vi "Command.vi"(8 "error in (no error)":errorcluster, 9 "data in":u8[](array[numeric]) format="%x", 10 "function code":u8=1 format="%x", 11 "MODBUS in":refnum<class "PL Modbus Client.lvclass">) -> (0 "error out":errorcluster, 2 "data out":u8[](array[numeric]) format="%x", 3 "MODBUS out":refnum<class "PL Modbus Client.lvclass">)   [LabVIEW 2015, in "PL Modbus Client.lvclass"]
doc: "Sends Modbus request with specified <B>function code</B> and <B>data in</B> and returns response data as <B>data out</B>. For not implemented function codes used via Modbus RTU <B>read RTU data callback</B> should be provided (default Read RTU Data.vi can be used as a template)."
uses:
  PL Modbus Client.lvclass
  PL Modbus Client.lvclass/PL Modbus Client.ctl
panel:
  out "exception":bool
  out "read buffer":string
  out "VISA locked":bool
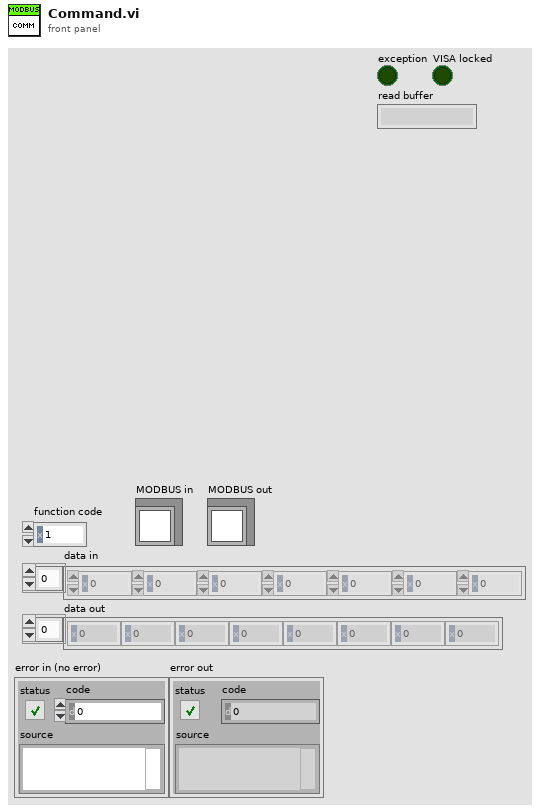
[diagram p1: front panel]
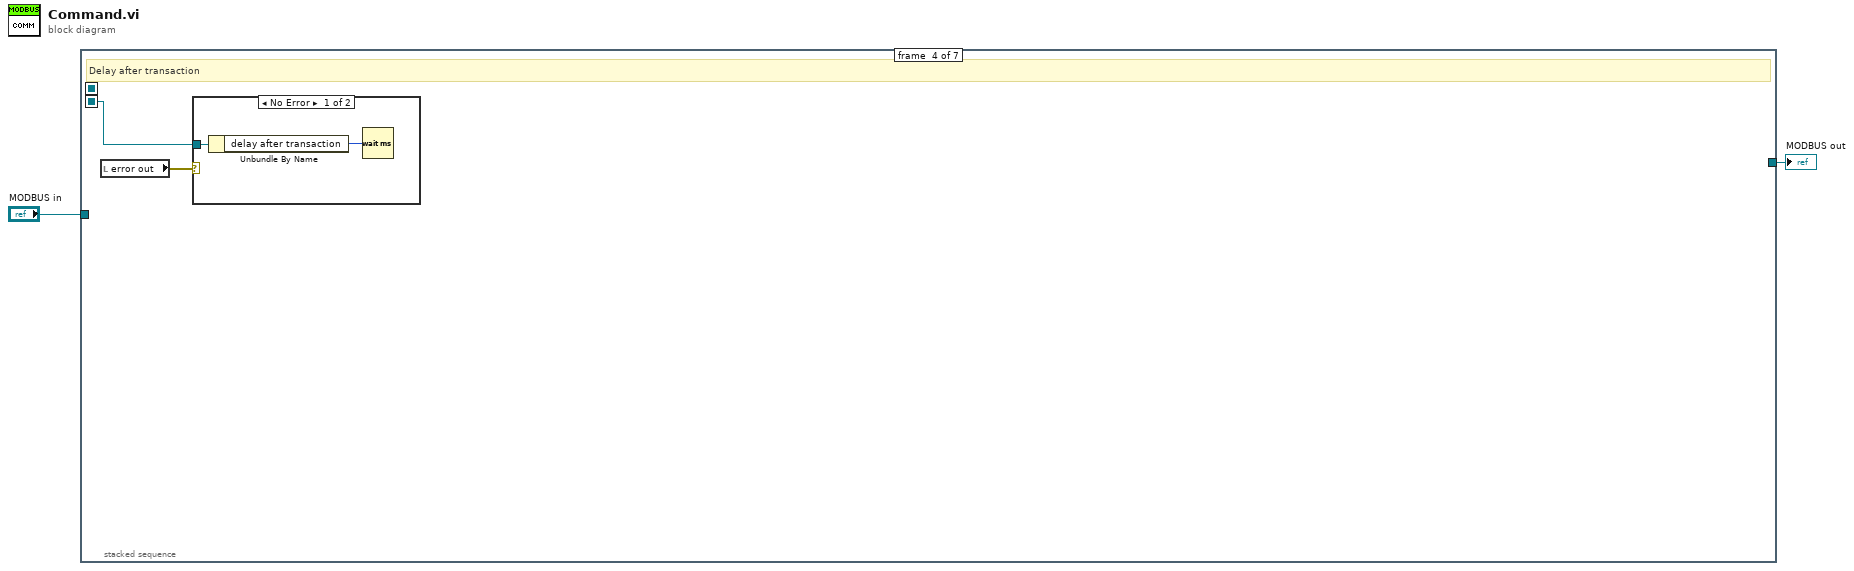
[diagram p0: block diagram]
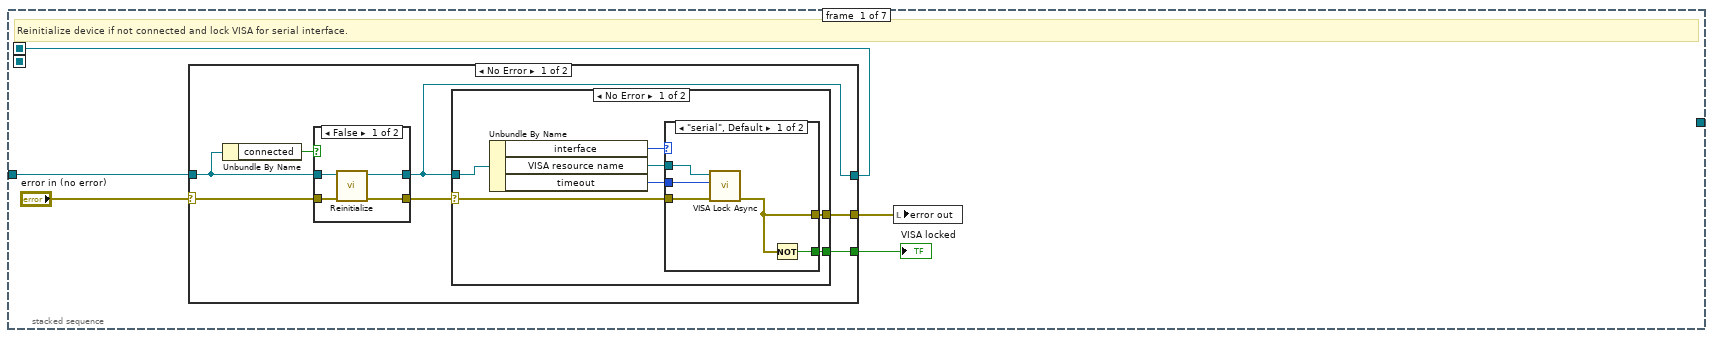
[diagram p2: hidden frame]
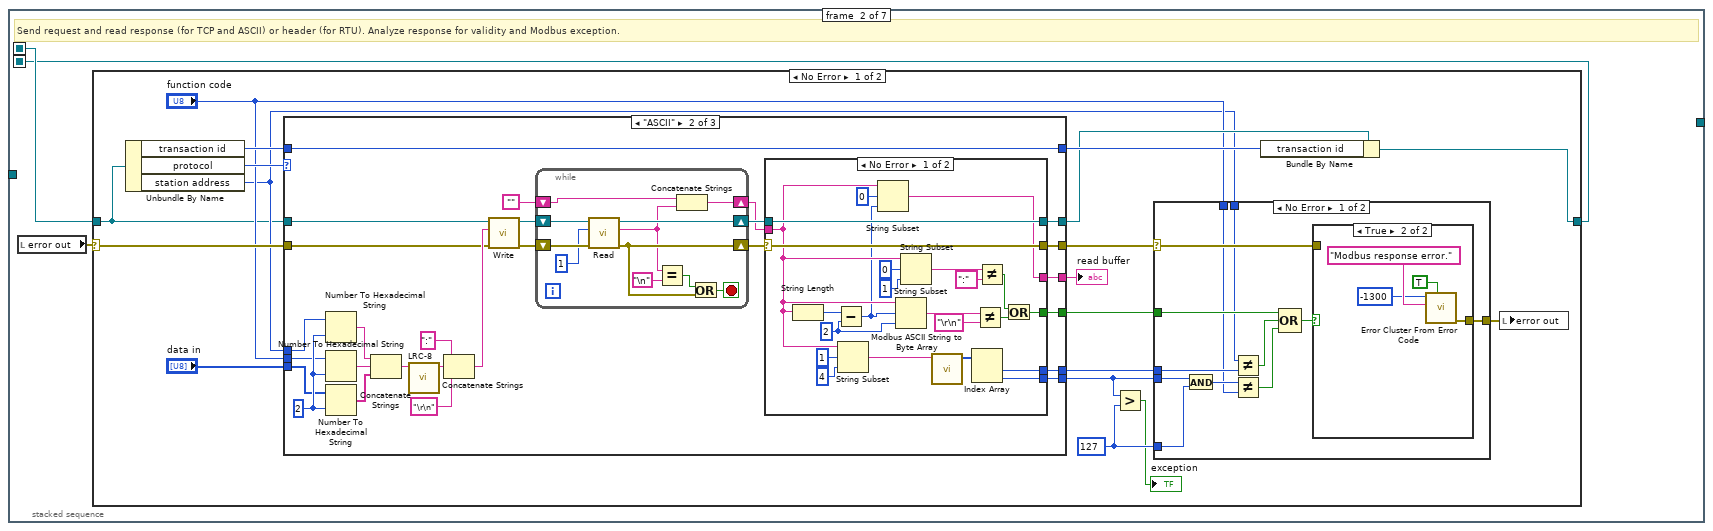
[diagram p7: hidden frame]
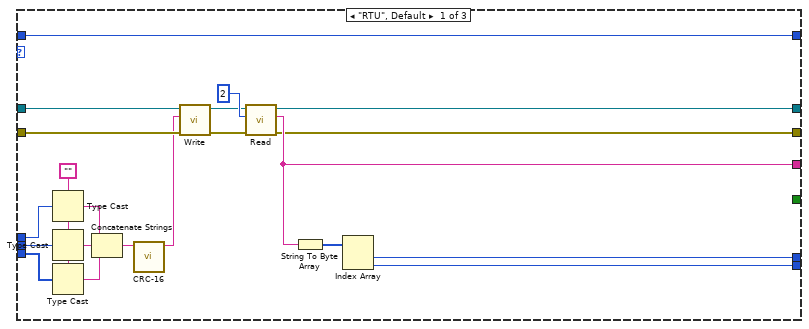
[diagram p10: hidden frame]
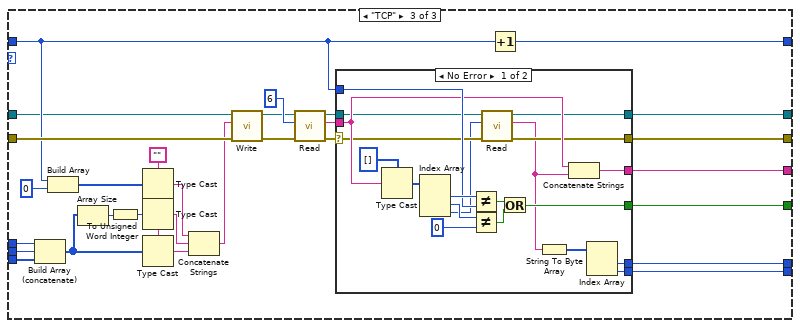
[diagram p12: hidden frame]
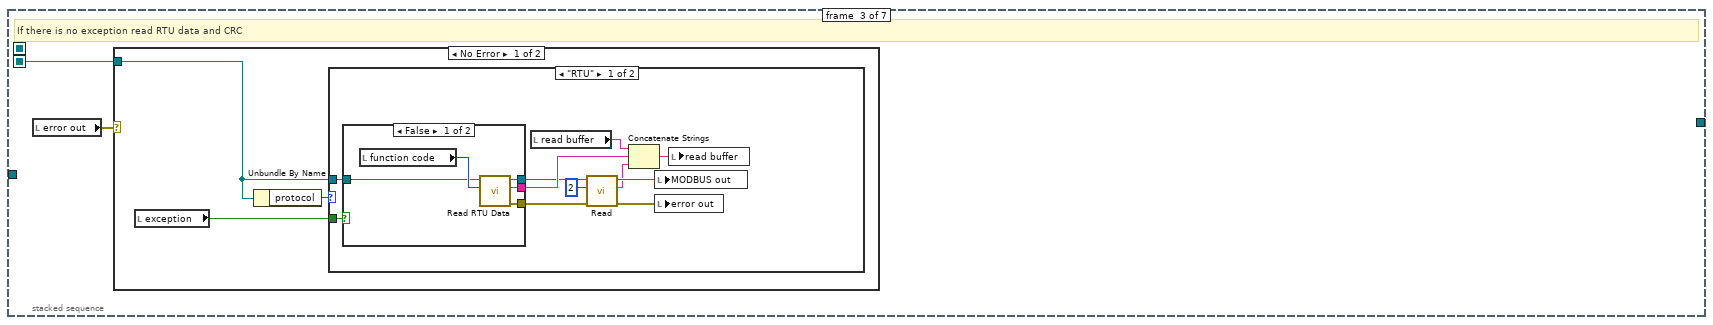
[diagram p15: hidden frame]
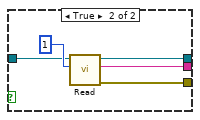
[diagram p16: hidden frame]
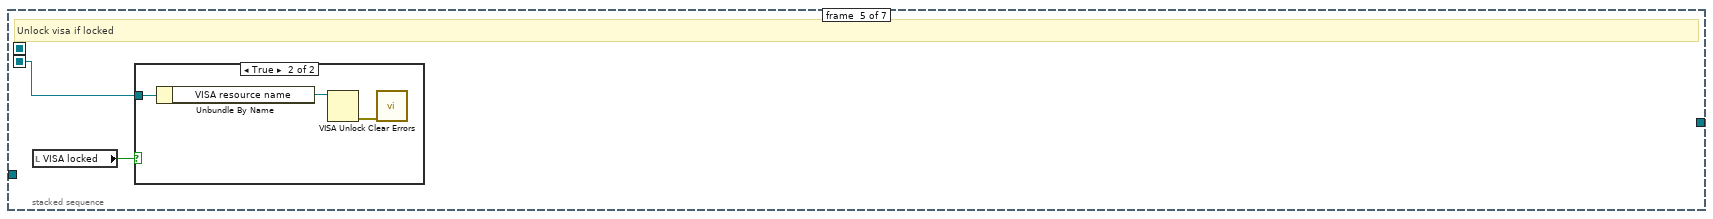
[diagram p20: hidden frame]
diagram:
  n1 = stacked-sequence {
    seq-local: [w4 _ _ _ _ _ _] -> [_ w38 _ _ _ _ _]
    seq-local: [_ w37 _ _ _ _ _] -> [_ _ w212 w239 w242 w247 w264]
    tunnel: [_ _ _ _ _ _ w263] -> w2
    tunnel: "MODBUS in" -> [w3 _ _ _ _ _ _]
    frame #0 {
      # "Reinitialize device if not connected and lock VISA for serial interface."
      n2 = case shown="No Error" "error in (no error)" {
        selector: "error in (no error)" -> [w9 w35]
        tunnel: [w14 _] -> w7
        tunnel: [w13 w35] -> w6
        tunnel: w3 -> [w11 w36]
        tunnel: [w8 w36] -> w4
        frame No Error {
          n3 = Unbundle By Name(w11) -> ("connected"=w12:bool)
          n4 = case shown="False" w12 {
            tunnel: w11 -> [w18 w20]
            tunnel: [w17 w20] -> w8
            tunnel: w9 -> [w15 w19]
            tunnel: [w16 w19] -> w10
            frame False {
              n5 = call "Reinitialize.vi"("error in (no error)"=w15, "MODBUS in"=w18) -> ("error out"=w16:errorcluster, "MODBUS out"=w17:refnum<class "PL Modbus Client.lvclass">)  [unwired: 8 in]
            }
            frame True {
            }
          }
          n6 = case shown="No Error" w10 {
            selector: w10 -> [w21 w34]
            tunnel: w8 -> [w26 _]
            tunnel: [w23 _] -> w14
            tunnel: [w22 w34] -> w13
            frame No Error {
              n7 = Unbundle By Name(w26) -> ("interface"=w27:enum16{"serial", "network"}, "VISA resource name"=w25:refnum<visa-resource-name>, "timeout"=w24:u32)
              n8 = case shown="\"serial\", Default" w27 {
                tunnel: w25 -> [w32 _]
                tunnel: w24 -> [w31 _]
                tunnel: [w30 _] -> w23
                tunnel: [w29 w33] -> w22
                tunnel: w21 -> [w28 w33]
                frame "serial", Default {
                  n9 = call <vilib>:"VISA Lock Async.vi"("error in (no error)"=w28, "timeout (0)"=w31, "VISA resource name"=w32) -> ("error out"=w29:errorcluster)  [unwired: 6 in, 2 out]
                  n10 = Not(x=w29) -> (.not. x?=w30:bool)
                }
                frame "network" {
                }
              }
            }
            frame Error {
            }
          }
        }
        frame Error {
        }
      }
      "VISA locked" <- w7
      n11 = local write "error out"(w6) -> ()
    }
    frame #1 {
      # "Send request and read response (for TCP and ASCII) or header (for RTU). Analyze response for validity and Modbus exception."
      n12 = local read "error out"() -> (w39:errorcluster)
      n13 = case shown="No Error" w39 {
        selector: w39 -> [w47 _]
        tunnel: w38 -> [w41 w211]
        tunnel: [w40 w211] -> w37
        frame No Error {
          w51 = u8 127
          n14 = Unbundle By Name(w41) -> ("transaction id"=w56:u16, "protocol"=w46:enum16{"RTU", "ASCII", "TCP"}, "station address"=w42:u8)
          n15 = case shown="\"ASCII\"" w46 {
            tunnel: w47 -> [w80 w98 w166]
            tunnel: [w77 w122 w187] -> w55
            tunnel: [w92 w113 w186] -> w45
            tunnel: [w96 w123 w188] -> w57
            tunnel: w56 -> [w96 w123 w161]
            tunnel: [w95 w119 w185] -> w53
            tunnel: [w94 w118 w184] -> w52
            tunnel: [_ w121 w183] -> w54
            tunnel: [w91 w120 w182] -> w48
            tunnel: w41 -> [w78 w97 w160]
            tunnel: "data in" -> [w82 w100 w168]
            tunnel: "function code" -> [w84 w102 w165]
            tunnel: w42 -> [w83 w101 w164]
            frame "RTU", Default {
              w85 = ""
              n16 = Type Cast(type=w85, x=w83) -> (*(type *) &x=w86:string)
              n17 = Type Cast(type=w85, x=w84) -> (*(type *) &x=w87:string)
              n18 = Type Cast(type=w85, x=w82) -> (*(type *) &x=w88:string)
              n19 = Concatenate Strings(w86, w87, w88) -> (w89:string)
              n20 = call "CRC-16.vi"("string"=w89) -> ("string with CRC-16"=w79:string)  [unwired: 9 in, 1 out]
              n21 = call "Write.vi"("error in (no error)"=w80, "write buffer"=w79, "MODBUS in"=w78) -> ("error out"=w76:errorcluster, "MODBUS out"=w81:refnum<class "PL Modbus Client.lvclass">)  [unwired: 7 in]
              n22 = call "Read.vi"("error in (no error)"=w76, "byte count"=u32 2, "MODBUS in"=w81) -> ("error out"=w77:errorcluster, "read buffer"=w91:string, "MODBUS out"=w92:refnum<class "PL Modbus Client.lvclass">)  [unwired: 6 in]
              n23 = String To Byte Array(string=w91) -> (unsigned byte array=w93:u8[])
              n24 = Index Array(array=w93) -> (element #1=w95:u8, element #2=w94:u8)  [unwired: 2 in]
            }
            frame "ASCII" {
              w106 = 2
              n25 = Number To Hexadecimal String(1:w106, 2:w101) -> (0:w110:string)
              n26 = Number To Hexadecimal String(1:w106, 2:w102) -> (0:w109:string)
              n27 = Number To Hexadecimal String(1:w106, 2:w100) -> (0:w103:string[])
              n28 = Concatenate Strings(w110, w109, w103) -> (w105:string)
              n29 = call "LRC-8.vi"("string"=w105) -> ("string with LRC-8"=w104:string)  [unwired: 9 in, 1 out]
              n30 = Concatenate Strings(":", w104, "\r\n") -> (w99:string)
              n31 = call "Write.vi"("error in (no error)"=w98, "write buffer"=w99, "MODBUS in"=w97) -> ("error out"=w111:errorcluster, "MODBUS out"=w112:refnum<class "PL Modbus Client.lvclass">)  [unwired: 7 in]
              n32 = while {
                shift-right: [w130] -> w117
                shift-left: w111 -> [w132]
                shift-right: [w133] -> w116
                shift-left: w112 -> [w134]
                shift-right: [w125] -> w114
                shift-left: "" -> [w124]
                stop <- w129 stop-if-true
                n33 = call "Read.vi"("error in (no error)"=w132, "byte count"=u32 1, "MODBUS in"=w134) -> ("error out"=w130:errorcluster, "read buffer"=w126:string, "MODBUS out"=w133:refnum<class "PL Modbus Client.lvclass">)  [unwired: 6 in]
                n34 = Equal?(x=w126, y="\n") -> (x = y?=w127:bool)
                n35 = Concatenate Strings(w124, w126) -> (w125:string)
                n36 = Or(x=w127, y=w130) -> (x .or. y?=w129:bool)
              }
              n37 = case shown="No Error" w117 {
                selector: w117 -> [w152 w159]
                tunnel: w116 -> [w156 w158]
                tunnel: [w152 w159] -> w122
                tunnel: [w156 w158] -> w113
                tunnel: w114 -> [w138 _]
                tunnel: [w142 _] -> w121
                tunnel: [w155 _] -> w119
                tunnel: [w154 _] -> w118
                tunnel: [w135 _] -> w120
                frame No Error {
                  w143 = 2 ("y")
                  n38 = String Length(string=w138) -> (length=w144:i32)
                  n39 = Subtract(x=w144, y=w143) -> (x-y=w136:i32)
                  n40 = String Subset(string=w138, offset (0)=1, length (rest)=4 ("length (rest)")) -> (substring=w145:string)
                  n41 = String Subset(string=w138, offset (0)=0, length (rest)=w136) -> (substring=w135:string)
                  n42 = String Subset(string=w138, offset (0)=w136, length (rest)=w143) -> (substring=w141:string)
                  n43 = String Subset(string=w138, offset (0)=0, length (rest)=1 ("length (rest)")) -> (substring=w150:string)
                  n44 = call "Modbus ASCII String to Byte Array.vi"("string"=w145) -> ("byte array"=w153:u8[])  [unwired: 10 in]
                  n45 = Index Array(array=w153) -> (element #1=w155:u8, element #2=w154:u8)  [unwired: 2 in]
                  n46 = Not Equal?(x=w141, y="\r\n") -> (x != y?=w140:bool)
                  n47 = Not Equal?(x=w150, y=":") -> (x != y?=w151:bool)
                  n48 = Or(x=w151, y=w140) -> (x .or. y?=w142:bool)
                }
                frame Error {
                }
              }
            }
            frame "TCP" {
              w172 = ""
              n49 = Build Array (concatenate)(w164, w165, w168) -> (w175:u8[])
              n50 = Build Array(w161, u16 0 ("element")) -> (w173:u16[])
              n51 = Array Size(array=w175) -> (size(s)=w176:i32)
              n52 = To Unsigned Word Integer(number=w176) -> (unsigned 16bit integer=w177:u16)
              n53 = Type Cast(type=w172, x=w173) -> (*(type *) &x=w174:string)
              n54 = Type Cast(type=w172, x=w177) -> (*(type *) &x=w169:string)
              n55 = Type Cast(type=w172, x=w175) -> (*(type *) &x=w170:string)
              n56 = Concatenate Strings(w174, w169, w170) -> (w162:string)
              n57 = call "Write.vi"("error in (no error)"=w166, "write buffer"=w162, "MODBUS in"=w160) -> ("error out"=w163:errorcluster, "MODBUS out"=w167:refnum<class "PL Modbus Client.lvclass">)  [unwired: 7 in]
              n58 = call "Read.vi"("error in (no error)"=w163, "byte count"=u32 6 ("bytes to read"), "MODBUS in"=w167) -> ("error out"=w181:errorcluster, "read buffer"=w178:string, "MODBUS out"=w179:refnum<class "PL Modbus Client.lvclass">)  [unwired: 6 in]
              n59 = case shown="No Error" w181 {
                selector: w181 -> [w193 w210]
                tunnel: [w192 w210] -> w187
                tunnel: w178 -> [w195 _]
                tunnel: w179 -> [w194 w209]
                tunnel: [w191 w209] -> w186
                tunnel: w161 -> [w202 _]
                tunnel: [w199 _] -> w185
                tunnel: [w198 _] -> w184
                tunnel: [w197 _] -> w183
                tunnel: [w196 _] -> w182
                frame No Error {
                  n60 = Type Cast(type=u16[] [], x=w195) -> (*(type *) &x=w207:u16[])
                  n61 = Index Array(array=w207) -> (element #1=w206:u16, element #2=w205:u16, element #3=w190:u16)  [unwired: 3 in]
                  n62 = Not Equal?(x=w206, y=w202) -> (x != y?=w201:bool)
                  n63 = Not Equal?(x=w205, y=u16 0) -> (x != y?=w200:bool)
                  n64 = call "Read.vi"("error in (no error)"=w193, "byte count"=w190, "MODBUS in"=w194) -> ("error out"=w192:errorcluster, "read buffer"=w189:string, "MODBUS out"=w191:refnum<class "PL Modbus Client.lvclass">)  [unwired: 6 in]
                  n65 = Or(x=w201, y=w200) -> (x .or. y?=w197:bool)
                  n66 = String To Byte Array(string=w189) -> (unsigned byte array=w203:u8[])
                  n67 = Concatenate Strings(w195, w189) -> (w196:string)
                  n68 = Index Array(array=w203) -> (element #1=w199:u8, element #2=w198:u8)  [unwired: 2 in]
                }
                frame Error {
                }
              }
              n69 = Increment(x=w161) -> (x+1=w188:u16)
            }
          }
          "read buffer" <- w48
          n70 = Greater?(x=w52, y=w51) -> (0:→"exception":bool)
          n71 = case shown="No Error" w55 {
            selector: w55 -> [w65 w75]
            tunnel: [w69 w75] -> w49
            tunnel: w54 -> [w64 _]
            tunnel: w53 -> [w61 _]
            tunnel: w52 -> [w60 _]
            tunnel: w42 -> [w59 _]
            tunnel: w51 -> [w67 _]
            tunnel: "function code" -> [w58 _]
            frame No Error {
              n72 = And(x=w60, y=w67) -> (x .and. y?=w66:u8)
              n73 = Not Equal?(x=w59, y=w61) -> (x != y?=w63:bool)
              n74 = Not Equal?(x=w66, y=w58) -> (x != y?=w62:bool)
              n75 = Compound Arithmetic op=OR(w64, w63, w62) -> (w68:bool)
              n76 = case shown="True" w68 {
                tunnel: [w70 w72] -> w69
                tunnel: w65 -> [w70 _]
                frame False {
                }
                frame True {
                  n77 = call <vilib>:"Error Cluster From Error Code.vi"("show call chain? (False)"=TRUE, "error message (\"\")"="Modbus response error." ("format string"), "error code (0)"=-1300) -> ("error out"=w72:errorcluster)  [unwired: 6 in]
                }
              }
            }
            frame Error {
            }
          }
          n78 = Bundle By Name(cluster=w45, "transaction id"=w57) -> (w40:refnum<class "PL Modbus Client.lvclass">)
          n79 = local write "error out"(w49) -> ()
        }
        frame Error {
        }
      }
    }
    frame #2 {
      # "If there is no exception read RTU data and CRC"
      n80 = local read "error out"() -> (w213:errorcluster)
      n81 = case shown="No Error" w213 {
        tunnel: w212 -> [w214 _]
        frame No Error {
          n82 = local read "exception"() -> (w216:bool)
          n83 = Unbundle By Name(w214) -> ("protocol"=w215:enum16{"RTU", "ASCII", "TCP"})
          n84 = case shown="\"RTU\"" w215 {
            tunnel: w214 -> [w227 _]
            tunnel: w216 -> [w226 _]
            frame "RTU" {
              n85 = case shown="False" w226 {
                tunnel: w227 -> [w231 w236]
                tunnel: [w230 w235] -> w222
                tunnel: [w229 w234] -> w221
                tunnel: [w228 w233] -> w223
                frame False {
                  n86 = local read "function code"() -> (w232:u8)
                  n87 = call-dynamic "Read RTU Data.vi"("function code"=w232, "MODBUS in"=w231) -> ("error out"=w229:errorcluster, "data"=w228:string, "MODBUS out"=w230:refnum<class "PL Modbus Client.lvclass">)  [unwired: 7 in]
                }
                frame True {
                  n88 = call "Read.vi"("byte count"=u32 1 ("data byte count"), "MODBUS in"=w236) -> ("error out"=w234:errorcluster, "read buffer"=w233:string, "MODBUS out"=w235:refnum<class "PL Modbus Client.lvclass">)  [unwired: 7 in]
                }
              }
              n89 = local read "read buffer"() -> (w225:string)
              n90 = call "Read.vi"("error in (no error)"=w221, "byte count"=u32 2 ("data byte count"), "MODBUS in"=w222) -> ("error out"=w218:errorcluster, "read buffer"=w217:string, "MODBUS out"=w219:refnum<class "PL Modbus Client.lvclass">)  [unwired: 6 in]
              n91 = Concatenate Strings(w225, w223, w217) -> (w224:string)
              n92 = local write "MODBUS out"(w219) -> ()
              n93 = local write "error out"(w218) -> ()
              n94 = local write "read buffer"(w224) -> ()
            }
            frame "ASCII", Default {
            }
          }
        }
        frame Error {
        }
      }
    }
    frame #3 {
      # "Delay after transaction"
      n95 = local read "error out"() -> (w238:errorcluster)
      n96 = case shown="No Error" w238 {
        tunnel: w239 -> [w241 _]
        frame No Error {
          n97 = Unbundle By Name(w241) -> ("delay after transaction"=w240:u32)
          n98 = Wait (ms)(milliseconds to wait=w240) -> ()  [unwired: 1 out]
        }
        frame Error {
        }
      }
    }
    frame #4 {
      # "Unlock visa if locked"
      n99 = local read "VISA locked"() -> (w243:bool)
      n100 = case shown="True" w243 {
        tunnel: w242 -> [_ w244]
        frame False {
        }
        frame True {
          n101 = Unbundle By Name(w244) -> ("VISA resource name"=w245:refnum<visa-resource-name>)
          n102 = VISA Unlock(11:w245) -> (0:w246:errorcluster)  [unwired: 1 in, 1 out]
          n103 = call <vilib>:"Clear Errors.vi"("error in (no error)"=w246) -> ()  [unwired: 5 in, 2 out]
        }
      }
    }
    frame #5 {
      # "Check CRC-16 (for RTU) or LRC-8 (for ASCII)"
      n104 = local read "error out"() -> (w248:errorcluster)
      n105 = case shown="No Error" w248 {
        tunnel: w247 -> [w249 _]
        frame No Error {
          n106 = Unbundle By Name(w249) -> ("protocol"=w252:enum16{"RTU", "ASCII", "TCP"})
          n107 = case shown="\"RTU\", Default" w252 {
            tunnel: [w255 w256 _] -> w250
            frame "RTU", Default {
              n108 = local read "read buffer"() -> (w254:string)
              n109 = call "CRC-16.vi"("string"=w254) -> ("CRC-16"=w253:u16)  [unwired: 9 in, 1 out]
              n110 = Not Equal To 0?(x=w253) -> (x != 0?=w255:bool)
            }
            frame "ASCII" {
              n111 = local read "read buffer"() -> (w257:string)
              n112 = call "LRC-8.vi"("string"=w257) -> ("LRC-8"=w258:u8)  [unwired: 9 in, 1 out]
              n113 = Not Equal To 0?(x=w258) -> (x != 0?=w256:bool)
            }
            frame "TCP" {
            }
          }
          n114 = case shown="True" w250 {
            tunnel: [_ w260] -> w251
            frame False {
            }
            frame True {
              n115 = call <vilib>:"Error Cluster From Error Code.vi"("show call chain? (False)"=TRUE, "error message (\"\")"="Modbus CRC error." ("format string"), "error code (0)"=-1300) -> ("error out"=w260:errorcluster)  [unwired: 6 in]
            }
          }
          n116 = local write "error out"(w251) -> ()
        }
        frame Error {
        }
      }
    }
    frame #6 {
      # "Convert data to U8 / Create Modbus exception error cluster / Set client state as \"not connected\""
      n117 = local read "error out"() -> (w265:errorcluster)
      n118 = case shown="No Error" w265 {
        selector: w265 -> [_ w312]
        tunnel: w264 -> [w266 w311]
        tunnel: [w266 w309] -> w263
        frame No Error {
          n119 = local read "read buffer"() -> (w271:string)
          n120 = Unbundle By Name(w266) -> ("protocol"=w267:enum16{"RTU", "ASCII", "TCP"})
          n121 = case shown="\"TCP\"" w267 {
            tunnel: w271 -> [w294 w301 w303]
            tunnel: [w293 w300 w302] -> w269
            frame "RTU", Default {
              n122 = String To Byte Array(string=w294) -> (unsigned byte array=w291:u8[])
              n123 = Array Size(array=w291) -> (size(s)=w290:i32)
              n124 = Subtract(x=w290, y=4) -> (x-y=w289:i32)
              n125 = Array Subset(array=w291, index=2, length=w289) -> (w293:u8[])
            }
            frame "ASCII" {
              n126 = String Length(string=w301) -> (length=w299:i32)
              n127 = Subtract(x=w299, y=7) -> (x-y=w297:i32)
              n128 = String Subset(string=w301, offset (0)=5, length (rest)=w297) -> (substring=w295:string)
              n129 = call "Modbus ASCII String to Byte Array.vi"("string"=w295) -> ("byte array"=w300:u8[])  [unwired: 10 in]
            }
            frame "TCP" {
              n130 = String To Byte Array(string=w303) -> (unsigned byte array=w307:u8[])
              n131 = Array Size(array=w307) -> (size(s)=w306:i32)
              n132 = Subtract(x=w306, y=8) -> (x-y=w305:i32)
              n133 = Array Subset(array=w307, index=8, length=w305) -> (w302:u8[])
            }
          }
          n134 = local read "exception"() -> (w270:bool)
          n135 = case shown="True" w270 {
            tunnel: w269 -> [w272 w287]
            tunnel: [w272 _] -> w268
            frame False {
            }
            frame True {
              w282 = ""
              n136 = Index Array(array=w287) -> (element=w274:u8)  [unwired: 1 in]
              n137 = Index Array(array=string[] ["", "ILLEGAL FUNCTION", "ILLEGAL DATA ADDRESS", "ILLEGAL DATA VALUE", "SERVER DEVICE FAILURE", "ACKNOWLEDGE", "SERVER DEVICE BUSY", "", "MEMORY PARITY ERROR", "", "GATEWAY PATH UNAVAILABLE", "GATEWAY TARGET DEVICE FAILED TO RESPOND"], index=w274) -> (element=w279:string)
              n138 = Not Equal?(x=w279, y=w282) -> (x != y?=w283:bool)
              n139 = Concatenate Strings(" (" ("string"), w279, ")" ("string")) -> (w278:string)
              n140 = Select(t=w278, s=w283, f=w282) -> (s? t:f=w276:string)
              n141 = Format Into String(format string="Modbus exception code 0x%02x%s.", w274, w276) -> (resulting string=w284:string)  [unwired: 2 in, 1 out]
              n142 = call <vilib>:"Error Cluster From Error Code.vi"("show call chain? (False)"=TRUE, "error message (\"\")"=w284, "error code (0)"=-1300) -> ("error out"=w273:errorcluster)  [unwired: 6 in]
              n143 = local write "error out"(w273) -> ()
            }
          }
          "data out" <- w268
        }
        frame Error {
          n144 = Unbundle By Name(w312) -> ("code"=w314:i32)
          n145 = Not Equal?(x=w314, y=-1300 ("error code (0)")) -> (x != y?=w313:bool)
          n146 = And(x=w312, y=w313) -> (x .and. y?=w310:bool)
          n147 = case shown="True" w310 {
            tunnel: w311 -> [w316 w319]
            tunnel: [w316 w317] -> w309
            frame False {
            }
            frame True {
              n148 = Bundle By Name(cluster=w319, "connected"=FALSE) -> (w317:refnum<class "PL Modbus Client.lvclass">)
            }
          }
        }
      }
    }
  }
  "MODBUS out" <- w2
